vi "LIA_FPGA.vi"() -> ()   [LabVIEW 2009]
uses:
  <vilib>/rvi/LocalResourceManager/LocalResourceManager.xnode
  <vilib>/rvi/eio/common/nirviEmuReportErrorAndStop.vi
  <vilib>/rvi/DataTransferAndStorage/Container/Common/niFpgaContainerSetEmuInfo.vi
  <vilib>/rvi/DataTransferAndStorage/Container/Common/niFpgaContainerState.ctl
  <vilib>/rvi/DataTransferAndStorage/Container/Common/niFpgaDataTypeControl.ctl
  <vilib>/rvi/DataTransferAndStorage/Container/Common/niFpgaContainerImplementationControl.ctl
  <vilib>/rvi/DataTransferAndStorage/Container/Common/niFpgaContainerArbitrationOptionsControl.ctl
  <vilib>/rvi/DataTransferAndStorage/Container/Common/niFpgaTransferTypeControl.ctl
  <vilib>/rvi/DataTransferAndStorage/Container/Common/niFpgaContainerInitializationParameters.ctl
  <vilib>/rvi/DataTransferAndStorage/Container/Common/niFpgaContainerMetaDataKey.ctl
  <vilib>/Platform/TimedLoop/XDataNode/XDataNode.xnode
  <vilib>/Platform/TimedLoop/XDataNode/loadlvalarms.vi
  <vilib>/Platform/TimedLoop/XDataNode/timing_clust.ctl
  <vilib>/Platform/TimedLoop/XDataNode/nitl_modes.ctl
  <vilib>/Platform/TimedLoop/XDataNode/wakeup.ctl
  <vilib>/rvi/DataTransferAndStorage/Container/XNode/niFpgaContainer.xnode
  <vilib>/rvi/FIFO/Fifo_Resource/nirvififoUniquifyingName.vi
  <vilib>/Platform/TimedLoop/XDataNode/XDNodeRunTimeDep.lvlib
panel:
  in  "Period":u16=1000
  out "ticks":u16
  out "ref":i16 format="%.0x"
  out "sig":i16 format="%.0x"
  out "channelQ":i64
  out "channelI":i64
  out "f":fxp<+/-,32,0> format="%.32g"
  in  "start":bool
  in  "dec2":i16=1
  in  "K":fxp<+,16,0>=0.001007080078125
  in  "nominal freq":fxp<+,16,0>=0.010009765625
  in  "dec1":i16=1
  in  "stages":i8=1
  in  "stop":bool
  in  "decimation":i16=1024
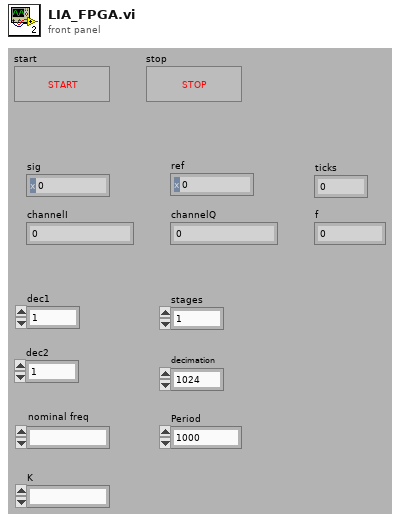
[diagram p1: front panel]
types:
  T1 = typedef "XDNodeRunTimeDep.lvlib/timing_clust.ctl" = cluster{"Expected End [f-1]":u64, "Actual End [f-1]":u64, "Finished Late? [f-1]":bool, "Expected End [i-1]":u64, "Actual End [i-1]":u64, "Finished Late? [i-1]":bool, "Expected Start [i]":u64, "Actual Start [i]":u64, "Expected Start [f]":u64, "Actual Start [f]":u64, "Source Name":string, "Structure Name":string, "Period":i64, "Deadline":i64, "Offset":i64, "Start":i64, "Priority":i32, "Timeout":i32, "Mode":T2, "Wakeup Reason":T3, "Error":errorcluster, "Source Type":string, "Secondary Source Type":string, "Global End Time":u64, "Global Start Time":u64, "Frame Duration":u64, "Iteration Duration":u64, "Assigned CPU":i32, "I/O Scan Engine Mode":u32}
  T2 = typedef "XDNodeRunTimeDep.lvlib/nitl_modes.ctl" = enum32{"No Change", "Process missed periods, maintain original phase", "Discard missed periods, maintain original phase", "Process missed periods, ignore original phase", "Discard missed periods, ignore original phase"}
  T3 = typedef "XDNodeRunTimeDep.lvlib/wakeup.ctl" = enum32{"Normal", "Aborted", "Asynchronous wakeup", "Timing source error", "Timed loop error", "Timeout"}
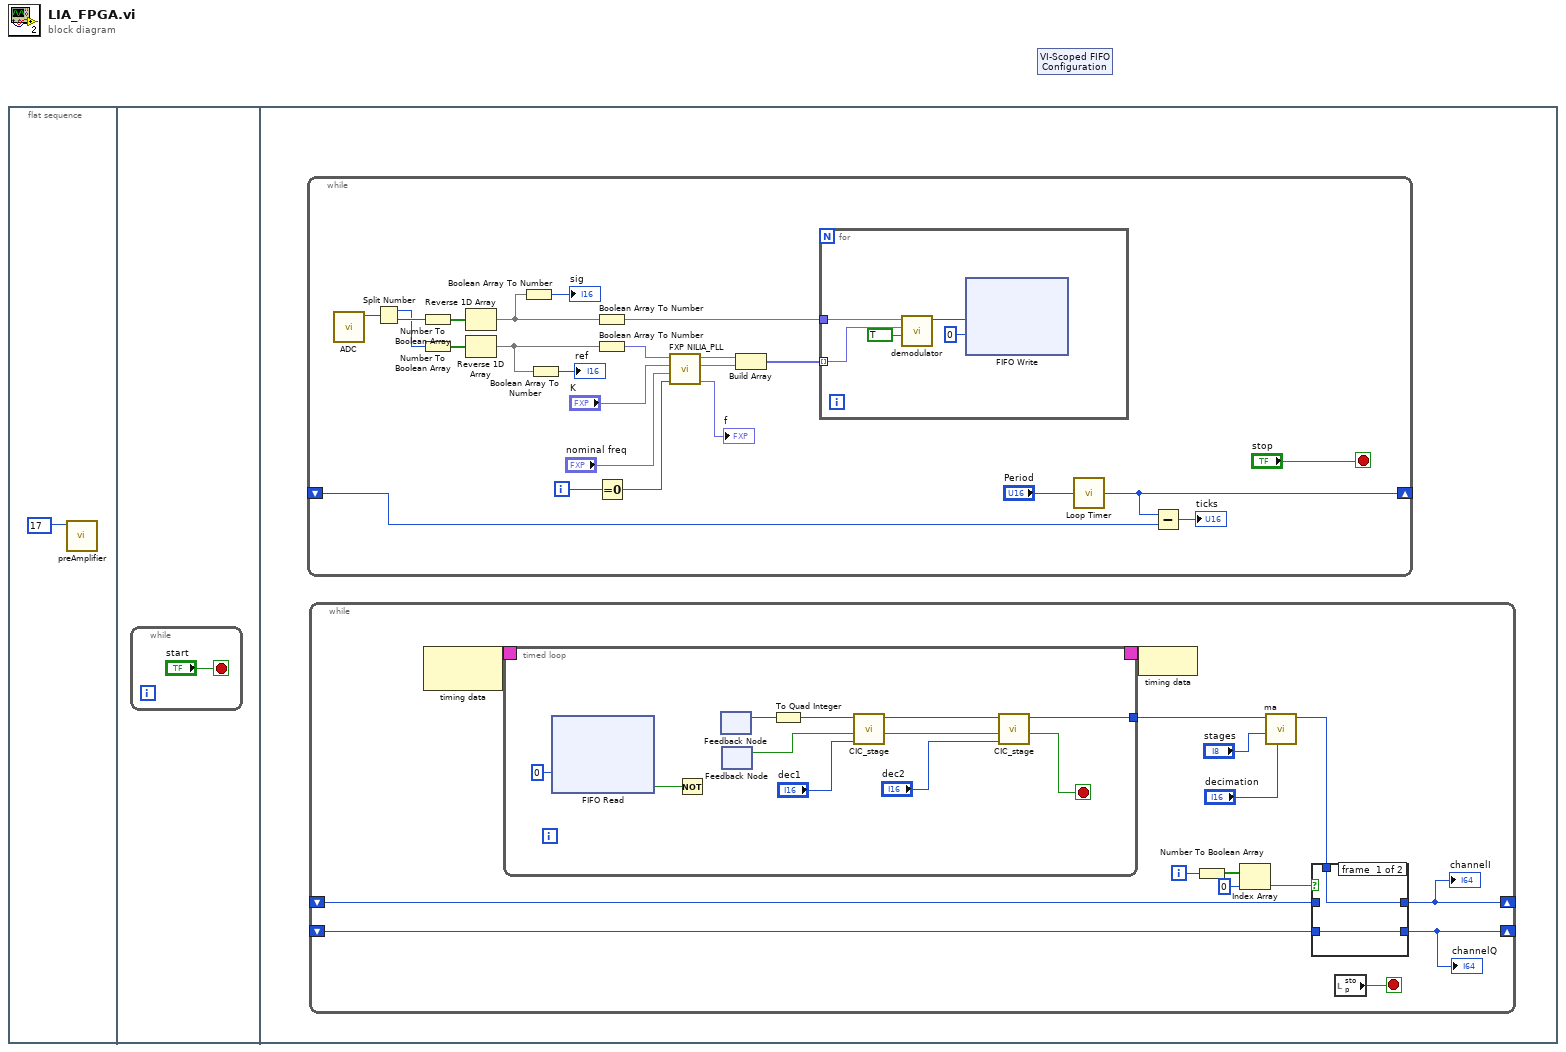
[diagram p0: block diagram]
diagram:
  n1 = flat-sequence {
    frame #0 {
      n2 = call "preAmplifier.vi"("Pre Code"=u8 17 ("PreAmplify")) -> ()  [unwired: 11 out]
    }
    frame #1 {
      n3 = while {
        stop <- "start" stop-if-true
      }
    }
    frame #2 {
      n4 = while {
        shift-right: [w13] -> _
        shift-left: _ -> [w12]
        i -> [w26]
        stop <- "stop" stop-if-true
        n5 = call "ADC.vi"() -> ("Output"=w17:u32)  [unwired: 1 in, 10 out]
        n6 = Split Number(x=w17) -> (hi(x)=w3:u16, lo(x)=w4:u16)
        n7 = Number To Boolean Array(number=w4) -> (Boolean array=w10:bool[])
        n8 = Number To Boolean Array(number=w3) -> (Boolean array=w9:bool[])
        n9 = Reverse 1D Array(array=w10) -> (reversed array=w8:bool[])
        n10 = Reverse 1D Array(array=w9) -> (reversed array=w6:bool[])
        n11 = Boolean Array To Number(Boolean array=w8) -> (number=→"sig":i16)
        n12 = Boolean Array To Number(Boolean array=w6) -> (number=→"ref":i16)
        n13 = Boolean Array To Number(Boolean array=w8) -> (number=w16:fxp<+/-,16,1>)
        n14 = Boolean Array To Number(Boolean array=w6) -> (number=w15:fxp<+/-,16,1>)
        n15 = Equal To 0?(x=w26) -> (x = 0?=w24:bool)
        n16 = call "FXP NILIA_PLL.vi"("reset?"=w24, "norminal freq [U16.0]"="nominal freq", "alpha [U16.0]"="K", "x[I16.1]"=w15) -> ("f"=→"f":fxp<+/-,32,0>, "sin(z)"=w19:fxp<+/-,16,2>, "cos(z)"=w20:fxp<+/-,16,2>)  [unwired: 1 in, 4 out]
        n17 = Build Array(w20, w19) -> (w18:fxp<+/-,16,2>[])
        n18 = for {
          tunnel: w16 -> [w28]
          tunnel: w18 -> [w27] mode=indexing
          n19 = call "demodulator.vi"("New Data"=TRUE, "ref"=w27, "signal"=w28) -> ("x*y"=w30:i32)  [unwired: 8 out]
          n20 = xnode ("FIFO Write")("Element"=w30, "Timeout"=0) -> ()  [unwired: 1 in, 2 out]
        }
        n21 = call "Loop Timer"("Count(Ticks)"="Period") -> ("Tick Count(Ticks)"=w13:u16)
        n22 = Subtract(x=w13, y=w12) -> (x-y=→"ticks":u16)
      }
      n23 = while {
        shift-right: [w81] -> _
        shift-left: _ -> [w83]
        shift-right: [w80] -> _
        shift-left: _ -> [w82]
        i -> [w88]
        stop <- w90 stop-if-true
        n24 = node-c288() -> (w94:T1)  [unwired: 1 out]
        n25 = timed-loop {
          timing: w94 -> [_]
          timing-out: [_] -> w93
          tunnel: [w102] -> w89
          stop <- w101 stop-if-true
          n26 = xnode ("FIFO Read")("Timeout"=0) -> ("Element"=w109:i32, "Timed Out?"=w108:bool)  [unwired: 1 in, 1 out]
          n27 = Not(x=w108) -> (.not. x?=w107:bool)
          n28 = feedback #1() -> (w111:i32)  [unwired: 1 out]
          n29 = feedback #2() -> (w105:bool)  [unwired: 1 out]
          n30 = To Quad Integer(1:w111) -> (0:w106:i64)
          n31 = call "CIC_stage.vi"("decimate factor"="dec1", "New Data"=w105, "input"=w106) -> ("Data Ready"=w103:bool, "output"=w104:i64)  [unwired: 7 out]
          n32 = call "CIC_stage.vi"("decimate factor"="dec2", "New Data"=w103, "input"=w104) -> ("Data Ready"=w101:bool, "output"=w102:i64)  [unwired: 7 out]
        }
        n33 = node-c288(w93) -> ()
        n34 = Number To Boolean Array(number=w88) -> (Boolean array=w87:bool[])
        n35 = Index Array(array=w87, index=0) -> (element=w85:bool)
        n36 = call "ma.vi"("decimate"="decimation", "stages"="stages", "input"=w89) -> ("output"=w84:i64)  [unwired: 8 out]
        n37 = case shown="True" w85 {
          tunnel: w84 -> [w96 w98]
          tunnel: [w96 w97] -> w81
          tunnel: [w95 w98] -> w80
          tunnel: w83 -> [_ w97]
          tunnel: w82 -> [w95 _]
          frame #0 {
          }
          frame #1 {
          }
        }
        "channelI" <- w81
        "channelQ" <- w80
        n38 = local read "stop"() -> (w90:bool)
      }
    }
  }
  n39 = xnode "VI-Scoped FIFO Configuration"() -> ()  [unwired: 1 out]
